vi "L1_fifttyIPRFinderNOPrint.vi"(0 "VISA In":refnum<visa-resource-name>="AgilentOsciloscope", 1 "Adder Register":i32=99, 2 "Vin":dbl=0.1, 3 "File path In":path=path "C:/Users/omartinez/Desktop/L0nL1_Results/L1_SN_00353_DT_Adder_Test.csv", 5 "ID In":refnum<k5>, 7 "Error In":errorcluster, 9 "Threshold Limits In":i16[](array[numeric])=[0, 512], 11 "Channel/Mode":i32=2, 12 "Adder Test?":bool=TRUE, 13 "Digital Output":i32=1) -> (4 "ID out":refnum<k5>, 6 "VISA Out":refnum<visa-resource-name>="AgilentOsciloscope", 10 "Threshold Limits Out":i16[](array[numeric])=[66, 67], 15 "Error Out":errorcluster)   [LabVIEW 2012]
uses:
  Sum_Abrilader/L0_Sum_Adder Folder/C/Program Files/National Instruments/LabVIEW 2012/instr.lib/Agilent 8000 Series/Public/Data/Low Level/Fetch Measurement (More).vi
  <vilib>/Utility/file.llb/Write To Spreadsheet File (DBL).vi
  <instrlib>/Agilent 8000 Series/Agilent 8000 Series.lvlib
panel:
  out "DAC Value":i32
  out "Current Threshold Limits Out":i16[](array[numeric])=[66, 67]
  out "Waveform Chart":dbl[](graph)
  in  "override control?":bool
  out "IPR_count 2":u32
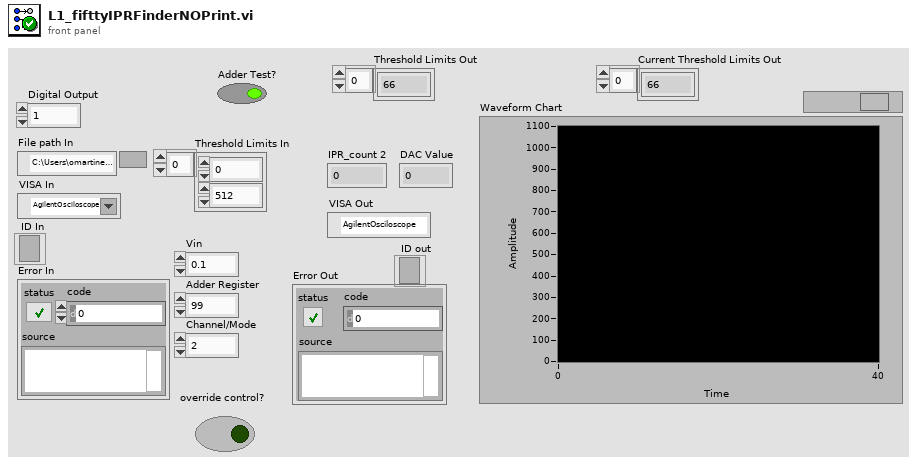
[diagram p1: front panel]
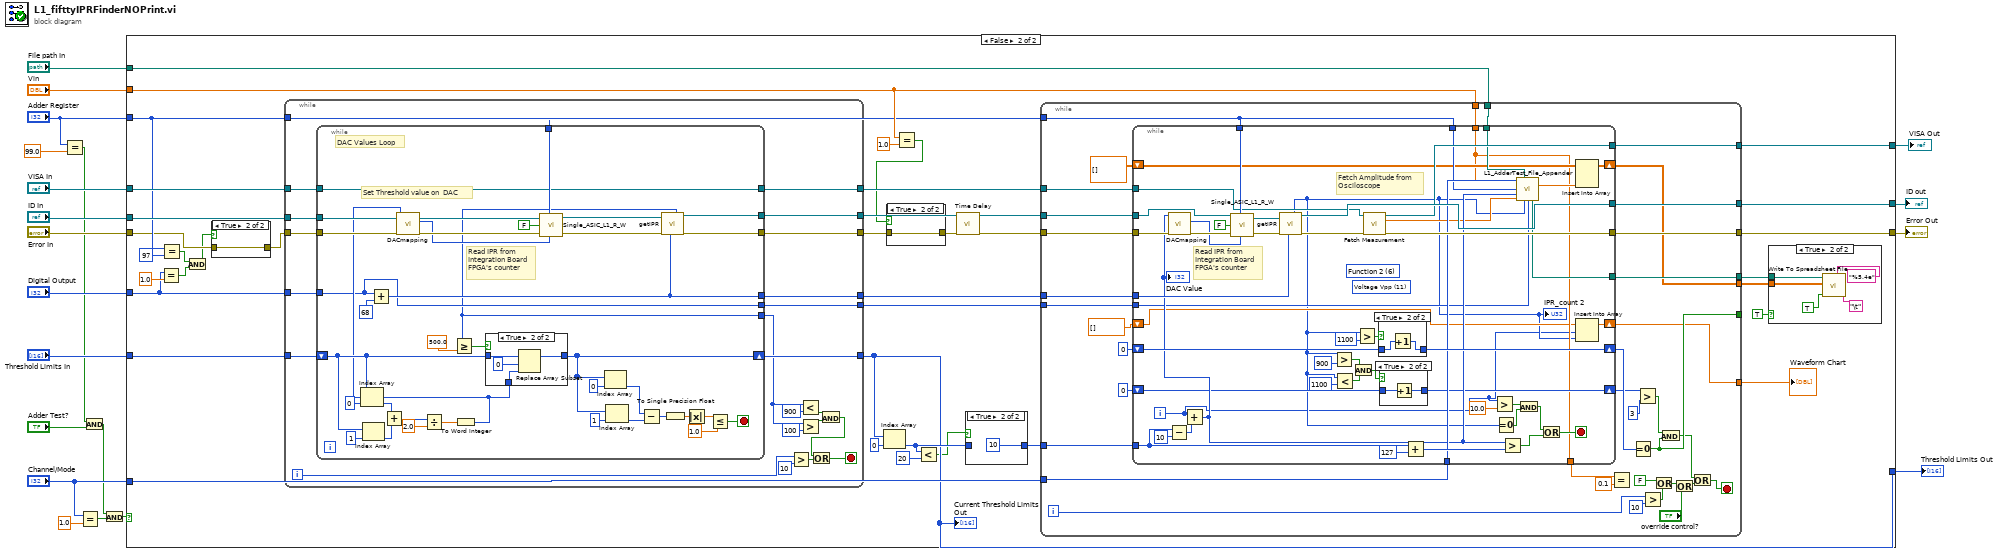
[diagram p0: block diagram]
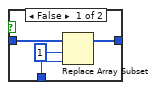
[diagram p6: hidden frame]
diagram:
  n1 = Equal?(x="Adder Register", y=99.0) -> (x = y?=w2:bool)
  n2 = Equal?(x="Channel/Mode", y=1.0) -> (x = y?=w8:bool)
  n3 = And(x=w2, y="Adder Test?") -> (x .and. y?=w1:bool)
  n4 = And(x=w1, y=w8) -> (x .and. y?=w9:bool)
  n5 = case shown="False" w9 {
    tunnel: "VISA In" -> [w24 w61]
    tunnel: "ID In" -> [w23 w60]
    tunnel: "Error In" -> [w22 w27]
    tunnel: "Threshold Limits In" -> [w21 w59]
    tunnel: "Digital Output" -> [_ w30]
    tunnel: [w22 w55] -> w15
    tunnel: "Vin" -> [_ w35]
    tunnel: "File path In" -> [_ w54]
    tunnel: [w23 w53] -> w12
    tunnel: "Adder Register" -> [_ w33]
    tunnel: [w21 w41] -> w11
    tunnel: "Channel/Mode" -> [_ w51]
    tunnel: [w24 w50] -> w10
    frame True {
    }
    frame False {
      n6 = Equal?(x=w30, y=1.0) -> (x = y?=w28:bool)
      n7 = Equal?(x=w33, y=97) -> (x = y?=w29:bool)
      n8 = And(x=w29, y=w28) -> (x .and. y?=w25:bool)
      n9 = case shown="True" w25 {
        tunnel: w27 -> [w62 w63]
        tunnel: [w62 w63] -> w26
        frame False {
        }
        frame True {
        }
      }
      n10 = while {
        tunnel: w61 -> [w89]
        tunnel: w60 -> [w88]
        tunnel: w26 -> [w87]
        tunnel: w59 -> [w86]
        tunnel: w30 -> [w85]
        tunnel: [w84] -> w37
        tunnel: [w83] -> w57
        tunnel: [w82] -> w56
        tunnel: w33 -> [w81]
        tunnel: [w80] -> w41
        tunnel: [w79] -> w52
        tunnel: [w78] -> w49
        i -> [w70]
        stop <- w71 stop-if-true
        n11 = while {
          tunnel: w88 -> [w125]
          tunnel: w81 -> [w123]
          tunnel: w87 -> [w122]
          tunnel: [w96] -> w84
          tunnel: w89 -> [w92]
          shift-right: [w100] -> w80
          shift-left: w86 -> [w104]
          tunnel: w85 -> [w91]
          tunnel: [w94] -> w83
          tunnel: [w93] -> w82
          tunnel: [w92] -> w79
          tunnel: [w91] -> w78
          tunnel: [w90] -> w75
          stop <- w103 stop-if-true
          # "Read IPR from \nIntegration Board\nFPGA's counter"
          # "Set Threshold value on  DAC"
          # "DAC Values Loop"
          n12 = Index Array(array=w104, index=0) -> (element=w110:i16)
          n13 = Index Array(array=w104, index=1) -> (element=w109:i16)
          n14 = Add(x=w91, y=68) -> (x+y=w93:i32)
          n15 = Add(x=w110, y=w109) -> (x+y=w115:i16)
          n16 = Divide(x=w115, y=2.0) -> (x/y=w111:dbl)
          n17 = To Word Integer(number=w111) -> (16bit integer=w95:i16)
          n18 = call "DACmapping.vi"("error in (no error)"=w122, "DAC_TH"=w95) -> ("error out"=w121:errorcluster, "COMB DEC"=w120:u32)  [unwired: 8 in]
          n19 = call "Single_ASIC_L1_R_W.vi"("connection ID"=w125, "Register or channel"=w123, "RD/#WR"=FALSE, "error in (no error)"=w121, "Data"=w120) -> ("connection ID out"=w118:refnum<k5>, "error out"=w119:errorcluster)  [unwired: 1 in, 2 out]
          n20 = call "getIPR.vi"("Address"=w93, "error in"=w119, "connection ID"=w118) -> ("error out"=w96:errorcluster, "connection ID out"=w94:refnum<k5>, "IPR_count"=w90:u32)  [unwired: 5 in, 1 out]
          n21 = Greater Or Equal?(x=w90, y=500.0) -> (x >= y?=w112:bool)
          n22 = case shown="True" w112 {
            tunnel: w104 -> [w127 w132]
            tunnel: [w126 w133] -> w100
            tunnel: w95 -> [w129 w130]
            frame False {
              n23 = Replace Array Subset(array=w127, new element=w129, index=1) -> (w126:i16[])
            }
            frame True {
              n24 = Replace Array Subset(array=w132, new element=w130, index=0) -> (w133:i16[])
            }
          }
          n25 = Index Array(array=w100, index=0) -> (element=w99:i16)
          n26 = Index Array(array=w100, index=1) -> (element=w98:i16)
          n27 = Subtract(x=w99, y=w98) -> (x-y=w108:i16)
          n28 = To Single Precision Float(number=w108) -> (single precision float=w107:sgl)
          n29 = Absolute Value(x=w107) -> (abs(x)=w106:sgl)
          n30 = Less Or Equal?(x=w106, y=sgl 1.0) -> (x <= y?=w103:bool)
        }
        n31 = Greater?(x=w70, y=10) -> (0:w68:bool)
        n32 = Less?(x=w75, y=u32 900) -> (x < y?=w77:bool)
        n33 = Greater?(x=w75, y=u32 100) -> (0:w76:bool)
        n34 = And(x=w77, y=w76) -> (x .and. y?=w72:bool)
        n35 = Or(x=w72, y=w68) -> (x .or. y?=w71:bool)
      }
      "Current Threshold Limits Out" <- w41
      n36 = Index Array(array=w41, index=0) -> (element=w43:i16)
      n37 = Equal?(x=w35, y=1.0) -> (x = y?=w38:bool)
      n38 = case shown="True" w38 {
        tunnel: w37 -> [w64 w65]
        tunnel: [w64 w65] -> w36
        frame False {
        }
        frame True {
        }
      }
      n39 = Less?(x=w43, y=i16 20) -> (x < y?=w40:bool)
      n40 = call "Time Delay"("error in (no error)"=w36) -> ("error out"=w45:errorcluster)  [unwired: 10 in]
      n41 = case shown="True" w40 {
        tunnel: w43 -> [w66 _]
        tunnel: [w66 i16 10] -> w44
        frame False {
        }
        frame True {
        }
      }
      n42 = while {
        tunnel: w44 -> [w174]
        tunnel: w45 -> [w173]
        tunnel: w57 -> [w172]
        tunnel: w56 -> [w171]
        tunnel: [w170] -> w55
        tunnel: w35 -> [w169]
        tunnel: w54 -> [w168]
        tunnel: [w167] -> w53
        tunnel: w33 -> [w166]
        tunnel: w52 -> [w165]
        tunnel: w51 -> [w164]
        tunnel: [w163] -> w50
        tunnel: w49 -> [w162]
        tunnel: [w159] -> w48
        tunnel: [w157] -> w47
        tunnel: [w140] -> w46
        tunnel: [w148] -> _
        i -> [w154]
        stop <- w155 stop-if-true
        n43 = while {
          tunnel: w174 -> [w223]
          tunnel: w173 -> [w215]
          tunnel: w172 -> [w214]
          tunnel: w171 -> [w213]
          tunnel: [w211] -> w170
          tunnel: w169 -> [w183]
          tunnel: w168 -> [w200]
          tunnel: w166 -> [w198]
          tunnel: [w210] -> w167
          tunnel: w166 -> [w209]
          tunnel: w165 -> [w208]
          tunnel: w164 -> [w199]
          tunnel: [w207] -> w163
          tunnel: w162 -> [w195]
          shift-right: [w201] -> w160
          shift-left: i16 0 ("y") -> [w202]
          tunnel: [w194] -> w159
          shift-right: [w192] -> w157
          shift-left: dbl[][] [] -> [w191]
          shift-right: [w184] -> w151
          shift-left: i16 0 ("y") -> [w185]
          tunnel: [w183] -> w144
          shift-right: [w178] -> w140
          shift-left: dbl[] [] -> [w177]
          i -> [w175]
          stop <- w206 stop-if-true
          (unwired) 11 items=["Rise Time", "Fall Time", "Frequency", "Period", "Voltage RMS(AC)", "Voltage RMS(DC)", "Voltage RMS (AC,cycle)", "Voltage RMS (DC,cycle)", "Voltage Max", "Voltage Min", "Voltage Middle", "Voltage Vpp", "Voltage High", "Voltage Low", "Voltage Average", "Voltage Average (cycle)", "Width Negative", "Width Positive", "Duty Cycle Positive", "Amplitude", "Overshoot", "Preshoot", "Voltage Base", "Voltage Upper", "Time Max", "Time Min", "Color Grade Crossing", "Color Grade Eye Width", "Color Grade Eye Height", "Color Grade Eye Q-Factory", "Color Grade Eye Duty Cycle Distortion(Percent)", "Color Grade Eye Duty Cycle Distortion(Time)", "Color Grade Eye Jitter(PP)", "Color Grade Eye Width(RMS)", "Cycle-cycle Duty Jitter(Rising)", "Cycle-cycle Duty Jitter(Falling)", "Cycle-cycle Jitter(Rising)", "Cycle-cycle Jitter(Falling)", "Cycle-cycle - Width", "Cycle-cycle + Width", "Date Rate", "Unit Interval", "FFT Delta Frequency", "FFT Delta Magnitude", "FFT Frequency", "FFT Magnitude", "Slew Rate", "Area (Entire Display)", "Area(Single Cycle)", "Duty Cycle (Rising)", "Duty Cycle (Falling)"] ("Measurement Function (0: Rise Time)")
          (unwired) 6 items=["Channel 1"=1, "Channel 2"=2, "Channel 3"=3, "Channel 4"=4, "Function 1"=5, "Function 2"=6, "Function 3"=7, "Function 4"=8, "Memory 1"=9, "Memory 2"=10, "Memory 3"=11, "Memory 4"=12] ("Channel (1: Channel 1)")
          # "Fetch Amplitude from\nOsciloscope"
          # "Read IPR from \nIntegration Board\nFPGA's counter"
          n44 = Subtract(x=w223, y=i16 10) -> (x-y=w221:i16)
          n45 = Add(x=w175, y=w221) -> (x+y=w197:i32)
          "DAC Value" <- w197
          n46 = call "DACmapping.vi"("error in (no error)"=w215, "DAC_TH"=w197) -> ("error out"=w219:errorcluster, "COMB DEC"=w218:u32)  [unwired: 8 in]
          n47 = call "Single_ASIC_L1_R_W.vi"("connection ID"=w214, "Register or channel"=w209, "RD/#WR"=FALSE, "error in (no error)"=w219, "Data"=w218) -> ("connection ID out"=w216:refnum<k5>, "error out"=w217:errorcluster)  [unwired: 1 in, 2 out]
          n48 = call "getIPR.vi"("Address"=w213, "error in"=w217, "connection ID"=w216) -> ("error out"=w212:errorcluster, "connection ID out"=w210:refnum<k5>, "IPR_count"=w176:u32)  [unwired: 5 in, 1 out]
          "IPR_count 2" <- w176
          n49 = Greater?(x=w176, y=u32 900) -> (0:w187:bool)
          n50 = Less?(x=w176, y=u32 1100) -> (x < y?=w188:bool)
          n51 = And(x=w187, y=w188) -> (x .and. y?=w186:bool)
          n52 = Greater?(x=w176, y=u32 1100) -> (0:w204:bool)
          n53 = call-poly "Fetch Measurement.vi"("VISA resource name"=w208, "error in (no error)"=w212) -> ("VISA resource name out"=w207:refnum<visa-resource-name>, "Measurement"=w196:dbl, "error out"=w211:errorcluster)  [unwired: 11 in]
          n54 = case shown="True" w204 {
            tunnel: w202 -> [w229 w231]
            tunnel: [w229 w230] -> w201
            frame False {
            }
            frame True {
              n55 = Increment(x=w231) -> (x+1=w230:i16)
            }
          }
          n56 = case shown="True" w186 {
            tunnel: [w226 w228] -> w184
            tunnel: w185 -> [w226 w227]
            frame False {
            }
            frame True {
              n57 = Increment(x=w227) -> (x+1=w228:i16)
            }
          }
          n58 = Add(x=w223, y=i16 127) -> (x+y=w225:i16)
          n59 = Greater?(x=w175, y=10.0) -> (0:w181:bool)
          n60 = Equal To 0?(x=w176) -> (x = 0?=w182:bool)
          n61 = Greater?(x=w197, y=w225) -> (0:w205:bool)
          n62 = call "L1_AdderTest_File_Appender.vi"("Vin"=w183, "file path (dialog if empty)"=w200, "CH"=w199, "Active Adder"=w198, "DAC Level"=w197, "Vmeas"=w196, "IPR"=w176, "Digital Output"=w195) -> ("appended array"=w193:dbl[], "file path (dialog if empty) 2"=w194:path)  [unwired: 6 in]
          n63 = And(x=w181, y=w182) -> (x .and. y?=w179:bool)
          n64 = Or(x=w179, y=w205) -> (x .or. y?=w206:bool)
          n65 = Insert Into Array(array=w191, new element=w193) -> (w192:dbl[][])  [unwired: 2 in]
          n66 = Insert Into Array(array=w177, index=w175, new element=w176) -> (w178:dbl[])
        }
        n67 = Equal?(x=w144, y=0.1) -> ()  [unwired: 1 out]
        n68 = Equal To 0?(x=w160) -> (x = 0?=w148:bool)
        n69 = Greater?(x=w151, y=i16 3) -> (0:w149:bool)
        n70 = Greater?(x=w154, y=10) -> (0:w156:bool)
        n71 = Or(x=FALSE, y=w156) -> (x .or. y?=w146:bool)
        n72 = And(x=w149, y=w148) -> (x .and. y?=w147:bool)
        n73 = Or(x=w146, y="override control?") -> (x .or. y?=w143:bool)
        n74 = Or(x=w147, y=w143) -> (x .or. y?=w155:bool)
      }
      "Waveform Chart" <- w46
      n75 = case shown="True" TRUE {
        tunnel: w48 -> [_ w137]
        tunnel: w47 -> [_ w136]
        frame False {
        }
        frame True {
          n76 = call-poly <vilib>:"Write To Spreadsheet File.vi"("delimiter (\\t)"="\t", "format (%.3f)"="%5.4e", "append to file? (new file:F)"=TRUE, "2D data"=w136, "file path (dialog if empty)"=w137) -> ()  [unwired: 3 in, 1 out]
        }
      }
    }
  }
  "Threshold Limits Out" <- w11
  "Error Out" <- w15
  "ID out" <- w12
  "VISA Out" <- w10
